vi "Controller Drive.vi"(0 "input cluster":T2) -> (14 "Strafe":dbl, 15 "Forward/Reverse":dbl, 16 "Turn":dbl, 17 "Picker Upper Up":bool, 18 "Picker Upper Down":bool)   [LabVIEW 2013]
uses:
  <vilib>/Rock Robotics/WPI/Joystick/WPI_JoystickButtonState.ctl
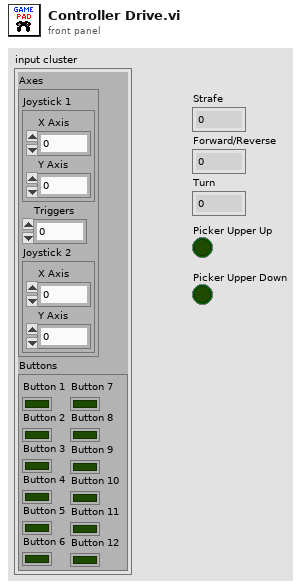
[diagram p1: front panel]
types:
  T1 = typedef "WPI_JoystickButtonState.ctl" = cluster{"Button 1":bool, "Button 2":bool, "Button 3":bool, "Button 4":bool, "Button 5":bool, "Button 6":bool, "Button 7":bool, "Button 8":bool, "Button 9":bool, "Button 10":bool, "Button 11":bool, "Button 12":bool}
  T2 = cluster{"Axes":cluster{"Joystick 1":cluster{"X Axis":dbl, "Y Axis":dbl}, "Triggers":dbl, "Joystick 2":cluster{"X Axis":dbl, "Y Axis":dbl}}, "Buttons":T1}
  T3 = cluster{"Joystick 1":cluster{"X Axis":dbl, "Y Axis":dbl}, "Triggers":dbl, "Joystick 2":cluster{"X Axis":dbl, "Y Axis":dbl}}
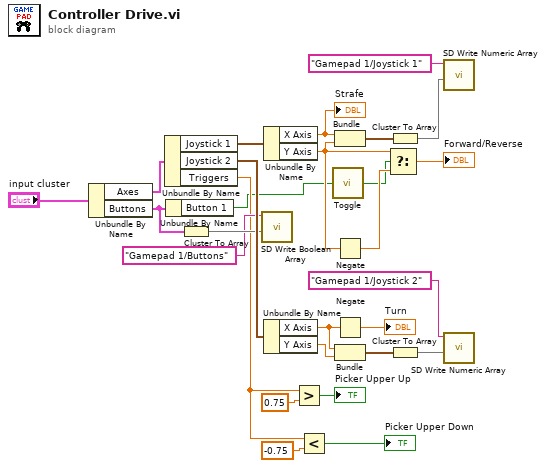
[diagram p0: block diagram]
diagram:
  n1 = Unbundle By Name("input cluster") -> ("Axes"=w27:T3, "Buttons"=w7:T1)
  n2 = Unbundle By Name(w27) -> ("Joystick 1"=w26:cluster{"X Axis":dbl, "Y Axis":dbl}, "Joystick 2"=w17:cluster{"X Axis":dbl, "Y Axis":dbl}, "Triggers"=w3:dbl)
  n3 = Unbundle By Name(w7) -> ("Button 1"=w2:bool)
  n4 = Cluster To Array(cluster=w7) -> (array=w9:bool[])
  n5 = call <vilib>:"SD Write Boolean Array.vi"("Boolean Array"=w9, "Name"="Gamepad 1/Buttons") -> ()  [unwired: 8 in, 2 out]
  n6 = Unbundle By Name(w26) -> ("X Axis"=w25:dbl, "Y Axis"=w14:dbl)
  "Strafe" <- w25
  n7 = Unbundle By Name(w17) -> ("X Axis"=w18:dbl, "Y Axis"=w20:dbl)
  n8 = Greater?(x=w3, y=0.75) -> (0:→"Picker Upper Up":bool)
  n9 = Less?(x=w3, y=-0.75) -> (x < y?=→"Picker Upper Down":bool)
  n10 = call "Toggle.vi"("Input"=w2) -> ("Latched"=w1:bool)
  n11 = Bundle("X Axis"=w25, "Y Axis"=w14) -> (w15:cluster{"X Axis":dbl, "Y Axis":dbl})  [unwired: 1 in]
  n12 = Negate(x=w14) -> (-x=w13:dbl)
  n13 = Negate(x=w18) -> (-x=→"Turn":dbl)
  n14 = Bundle("X Axis"=w18, "Y Axis"=w20) -> (w22:cluster{"X Axis":dbl, "Y Axis":dbl})  [unwired: 1 in]
  n15 = Select(t=w14, s=w1, f=w13) -> (s? t:f=→"Forward/Reverse":dbl)
  n16 = Cluster To Array(cluster=w15) -> (array=w24:dbl[])
  n17 = Cluster To Array(cluster=w22) -> (array=w21:dbl[])
  n18 = call <vilib>:"SD Write Numeric Array.vi"("Numeric Array"=w24, "Name"="Gamepad 1/Joystick 1") -> ()  [unwired: 8 in, 2 out]
  n19 = call <vilib>:"SD Write Numeric Array.vi"("Numeric Array"=w21, "Name"="Gamepad 1/Joystick 2") -> ()  [unwired: 8 in, 2 out]
